vi "rslcx_LV2015_Read_Device_IDN_Example.vi"() -> ()   [LabVIEW 2015]
uses:
  <instrlib>/Rohde&Schwarz LCX LCR Meter/Rohde&Schwarz LCX LCR Meter.lvlib
panel:
  out "*IDN? response":string
  in  "VISA resource name":refnum<visa-resource-name>="TCPIP::10.102.189.20::hislip0"
  in  "Reset":bool
  in  "ID Query":bool=TRUE
  # "Rohde & Schwarz LCR Meter\n*IDN? Example"
  # "Before running, change the VISA resource name to fit your device:\n- For LAN interface use TCPIP::<IP_Address>::INSTR e.g. TCPIP::10.64.0.178::INSTR\n- For USB interface use USB0::0x0AAD::<PID>::<SN>::INSTR e.g. USB0::0x0AAD::0x01D6::101457::INSTR\n- For GPIB interface use the GPIB::<Address>::INSTR e.g. GPIB::28::INSTR"
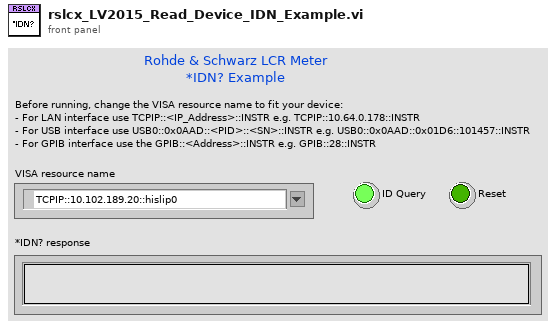
[diagram p1: front panel]
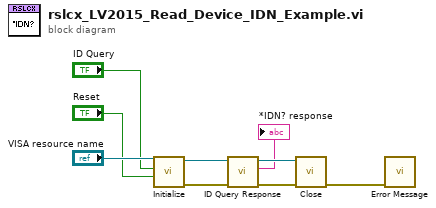
[diagram p0: block diagram]
diagram:
  n1 = call <instrlib>:"Initialize.vi"("Reset (T: Reset)"="Reset", "ID Query (T: Check)"="ID Query", "VISA resource name"="VISA resource name") -> ("error out"=w8:errorcluster, "VISA resource name out"=w7:refnum<visa-resource-name>)  [unwired: 7 in]
  n2 = call <instrlib>:"ID Query Response.vi"("error in (no error)"=w8, "VISA resource name"=w7) -> ("error out"=w6:errorcluster, "ID Query Response"=→"*IDN? response":string, "VISA resource name out"=w5:refnum<visa-resource-name>)  [unwired: 7 in]
  n3 = call <instrlib>:"Close.vi"("error in (no error)"=w6, "VISA resource name"=w5) -> ("error out"=w4:errorcluster)  [unwired: 9 in]
  n4 = call <instrlib>:"Error Message.vi"("error in (no error)"=w4) -> ()  [unwired: 10 in, 5 out]
